vi "Demo STLtoSVG.vi"(8 "File True/ String False":bool=TRUE, 9 "Scale":i32=50, 10 "STL String":string, 11 "file (use dialog)":path) -> (2 "new picture":picture)   [LabVIEW 2019]
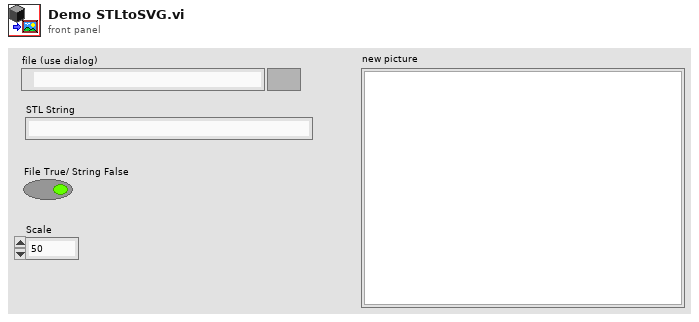
[diagram p1: front panel]
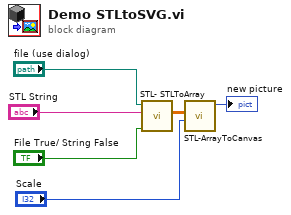
[diagram p0: block diagram]
diagram:
  n1 = call <userlib>:"STL- STLToArray.vi"("Boolean"="File True/ String False", "String"="STL String", "file (use dialog)"="file (use dialog)") -> ("Array 3"=w3:dbl[][])  [unwired: 8 in]
  n2 = call <userlib>:"STL-ArrayToCanvas.vi"("Scale"="Scale", "STL array"=w3) -> ("Picture Out"=→"new picture":picture)  [unwired: 9 in]
